vi "Read Device Identification1.vi"(8 "error in (no error)":errorcluster, 9 "object ID":u8, 10 "device ID category":T2(ring), 11 "Modbus master in":refnum<class "TCP.lvclass">) -> (0 "error out":errorcluster, 2 "objects":cluster{"object ID":u8, "value":string}[](array[cluster]) {"object ID" format="%x"}, 3 "Modbus master out":refnum<class "TCP.lvclass">)   [LabVIEW 2019, in "NI_modbus_upd.lvlib"]
doc: "Returns the device identification of a Modbus slave. Device identification consists of data elements called objects. Each object has an identification number and stores Modbus slave information."
uses:
  NI_modbus_upd.lvlib
  TCP/TCP.lvclass
  Ctl/Unit_ID.ctl
  TCP/TCP.lvclass/TCP.ctl
  Convert to String.vi
  Function code mismatch error1.vi
  Error Generator1.vi
  Modbus Data Unit (PDU)/Construct PDU1.vi
  Read ADU Packet Master.vi
  Write ADU Packet Master.vi
  Modbus Data Unit (PDU)/Unflatten to PDU1.vi
  TCP/Protocol Read.vi
  TCP/Protocol Write.vi
  <vilib>/Utility/error.llb/Error Cluster From Error Code.vi
  Modbus Data Unit (PDU)/Deconstruct PDU1.vi
panel:
  in  "Unit_ID":T1
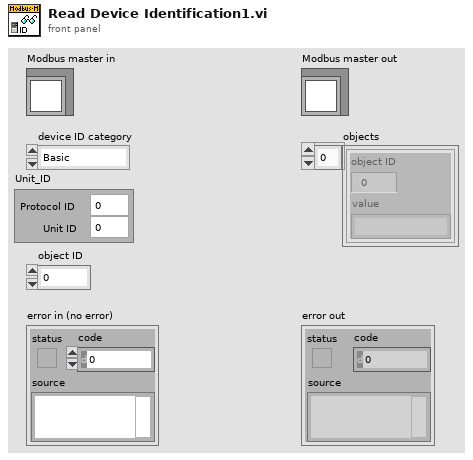
[diagram p1: front panel]
types:
  T1 = typedef "NI_modbus_upd.lvlib/Unit_ID.ctl" = cluster{"Protocol ID":u16, "Unit ID":u8}
  T2 = enum8{"Basic", "Regular", "Extended", "Specific"}
  T3 = typedef "NI_modbus_upd.lvlib/MB Modbus Data Unit.ctl" = cluster{"function":T4, "Data":u8[]}
  T4 = typedef "NI_modbus_upd.lvlib/Function.ctl" = u8
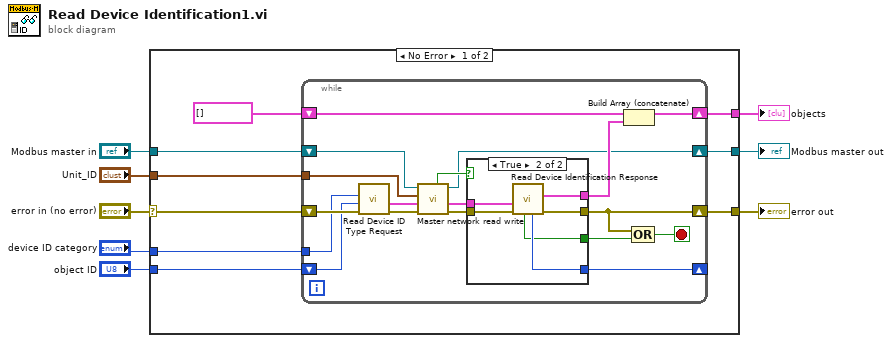
[diagram p0: block diagram]
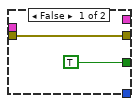
[diagram p2: hidden frame]
diagram:
  n1 = case shown="No Error" "error in (no error)" {
    selector: "error in (no error)" -> [w9 w45]
    tunnel: "Modbus master in" -> [w11 w44]
    tunnel: [w12 w44] -> w6
    tunnel: [w13 w45] -> w5
    tunnel: "device ID category" -> [w17 _]
    tunnel: "object ID" -> [w16 _]
    tunnel: [w15 _] -> w3
    tunnel: "Unit_ID" -> [w10 _]
    frame No Error {
      n2 = while {
        tunnel: w17 -> [w34]
        shift-right: [w31] -> w13
        shift-left: w9 -> [w35]
        shift-right: [w30] -> w15
        shift-left: cluster{"object ID":u8, "value":string}[] [] -> [w29]
        shift-right: [w28] -> _
        shift-left: w16 -> [w33]
        shift-right: [w19] -> w12
        shift-left: w11 -> [w22]
        tunnel: w10 -> [w20]
        stop <- w32 stop-if-true
        n3 = call "Read Device ID Type Request.vi"("error in (no error)"=w35, "object ID"=w33, "read device ID code"=w34) -> ("error out"=w24:errorcluster, "Modbus Data Unit out"=w21:T3)  [unwired: 7 in]
        n4 = call "Master network read write.vi"("error in (no error)"=w24, "Modbus Data Unit"=w21, "Unit_ID"=w20, "TCP in"=w22) -> ("error out"=w25:errorcluster, "Modbus data unit out"=w18:T3, "TCP out"=w19:refnum<class "TCP.lvclass">, "PDU valid?"=w23:bool)  [unwired: 4 in]
        n5 = case shown="True" w23 {
          tunnel: [w37 w43] -> w31
          tunnel: [_ w42] -> w28
          tunnel: [TRUE ("done?") w41] -> w27
          tunnel: [_ w40] -> w26
          tunnel: w25 -> [w37 w39]
          tunnel: w18 -> [_ w38]
          frame False {
          }
          frame True {
            n6 = call "Read Device Identification Response.vi"("error in (no error)"=w39, "Modbus Data Unit in"=w38) -> ("error out"=w43:errorcluster, "objects"=w40:cluster{"object ID":u8, "value":string}[], "next object ID"=w42:u8, "done?"=w41:bool)  [unwired: 5 in, 1 out]
          }
        }
        n7 = Build Array (concatenate)(w29, w26) -> (w30:cluster{"object ID":u8, "value":string}[])
        n8 = Compound Arithmetic op=OR(w31, w27) -> (w32:bool)
      }
    }
    frame Error {
    }
  }
  "error out" <- w5
  "Modbus master out" <- w6
  "objects" <- w3
